vi "Join StringsSD.vi"(1 "string array":string[](array[string]), 2 "delimiter (\"\")":string, 3 "right decoration (\"\")":string, 4 "left decoration (\"\")":string) -> (0 "joined string":string)   [LabVIEW 2015]
doc: "Joins an array of strings into one single string.\n\nThe resulting string is created by concatenating;\nleft_decoration + string_array[0] + right_decoration + delimiter +\nleft_decoration + string_array[1] + right_decoration + delimiter +\n... +\nleft_decoration + string_array[n] + right_decoration."
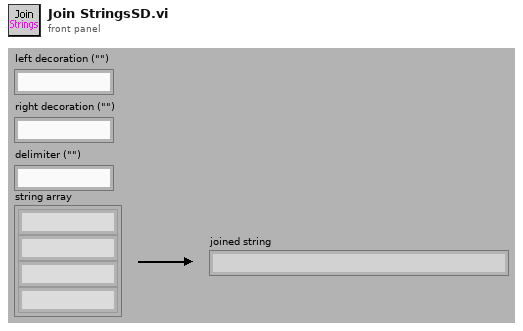
[diagram p1: front panel]
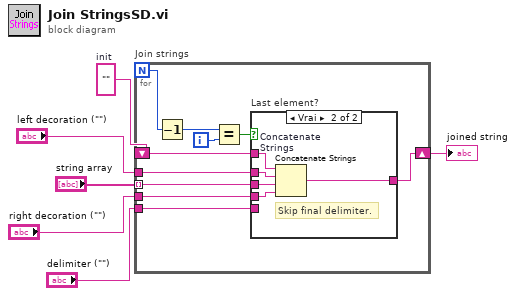
[diagram p0: block diagram]
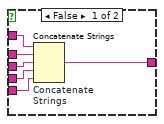
[diagram p2: hidden frame]
diagram:
  w6 = ""  # init
  n1 = for "Join strings" {
    N -> [w10]
    tunnel: "string array" -> [w14] mode=indexing
    shift-right: [w16] -> w1
    shift-left: w6 -> [w15]
    tunnel: "left decoration (\"\")" -> [w13]
    tunnel: "right decoration (\"\")" -> [w12]
    tunnel: "delimiter (\"\")" -> [w11]
    i -> [w8]
    n2 = Decrement(x=w10) -> (x-1=w9:i32)
    n3 = Equal?(x=w9, y=w8) -> (x = y?=w7:bool)
    n4 = case "Last element?" shown="Vrai" w7 {
      tunnel: [w22 w23] -> w16
      tunnel: w15 -> [w21 w27]
      tunnel: w14 -> [w20 w25]
      tunnel: w13 -> [w19 w26]
      tunnel: w12 -> [w18 w24]
      tunnel: w11 -> [w17 _]
      frame False {
        n5 = Concatenate Strings "Concatenate\nStrings"(w21, w19, w20, w18, w17) -> (w22:string)
      }
      frame True {
        # "Skip final delimiter."
        n6 = Concatenate Strings "Concatenate\nStrings"(w27, w26, w25, w24) -> (w23:string)
      }
    }
  }
  "joined string" <- w1
